vi "MXA_FSM_SweeptSA.vi"() -> ()   [LabVIEW 2021]
uses:
  MXA_TypeofMeasurment_Control.ctl
  MXA_FSM_Control.ctl
  <vilib>/Utility/error.llb/DialogType.ctl
  Control 2.ctl
  Control 3.ctl
  Control 4.ctl
  Keysight XSAn/Keysight XSAn.lvlib
panel:
  in  "ON/OFF TRIGGER":bool
  out "Power_in(mW) 2":dbl
  in  "Reset SA":bool
  out "Error SA":errorcluster
  out "Error Power Meter 2":errorcluster
  out "NewVal 2":bool
  out "Power_out(mW)":dbl
  out "Power Meter out":dbl[](graph)
  out "Power Meter Out":bool
  in  "Power Meter Out":refnum<visa-resource-name>="PM100D" caption="resource name"
  out "Power Meter in":dbl[](graph)
  in  "Power Meter In":refnum<visa-resource-name>="PM100D" caption="resource name"
  out "Power Meter In":bool
  in  "Reset Power Meter":bool
  out "Power_in(mW)":dbl
  out "NewVal":bool
  out "Error Power Meter":errorcluster
  in  "file (use dialog)":path
  in  "Base Name":string
  in  "ExternalTriggerLevel":dbl=1.0 caption="Ex_Trig_Level"
  out "Measurement Type":T1=enum."S-Meas"
  in  "Type of Normalization":enum32{"(S-N)/(N-E)", "(S-E)/(E)"}(radio)=enum."(S-E)/(E)"
  out "XY-Graph":cluster{"Val":dbl[], "Val":dbl[]}(graph)
  in  "S measurement":bool
  in  "N measurement":bool
  in  "E measurement":bool
  in  "Averages":i32
  in  "span":dbl=1000.0 caption="span (MHz)"
  in  "center frequency":dbl=520.0 caption="center frequency (MHz)"
  in  "Spectrum analyzer":string="TCPIP0::K-N9020B-50216::inst0::INSTR" caption="resource name"
  in  "stop":bool
  # "Triggering"
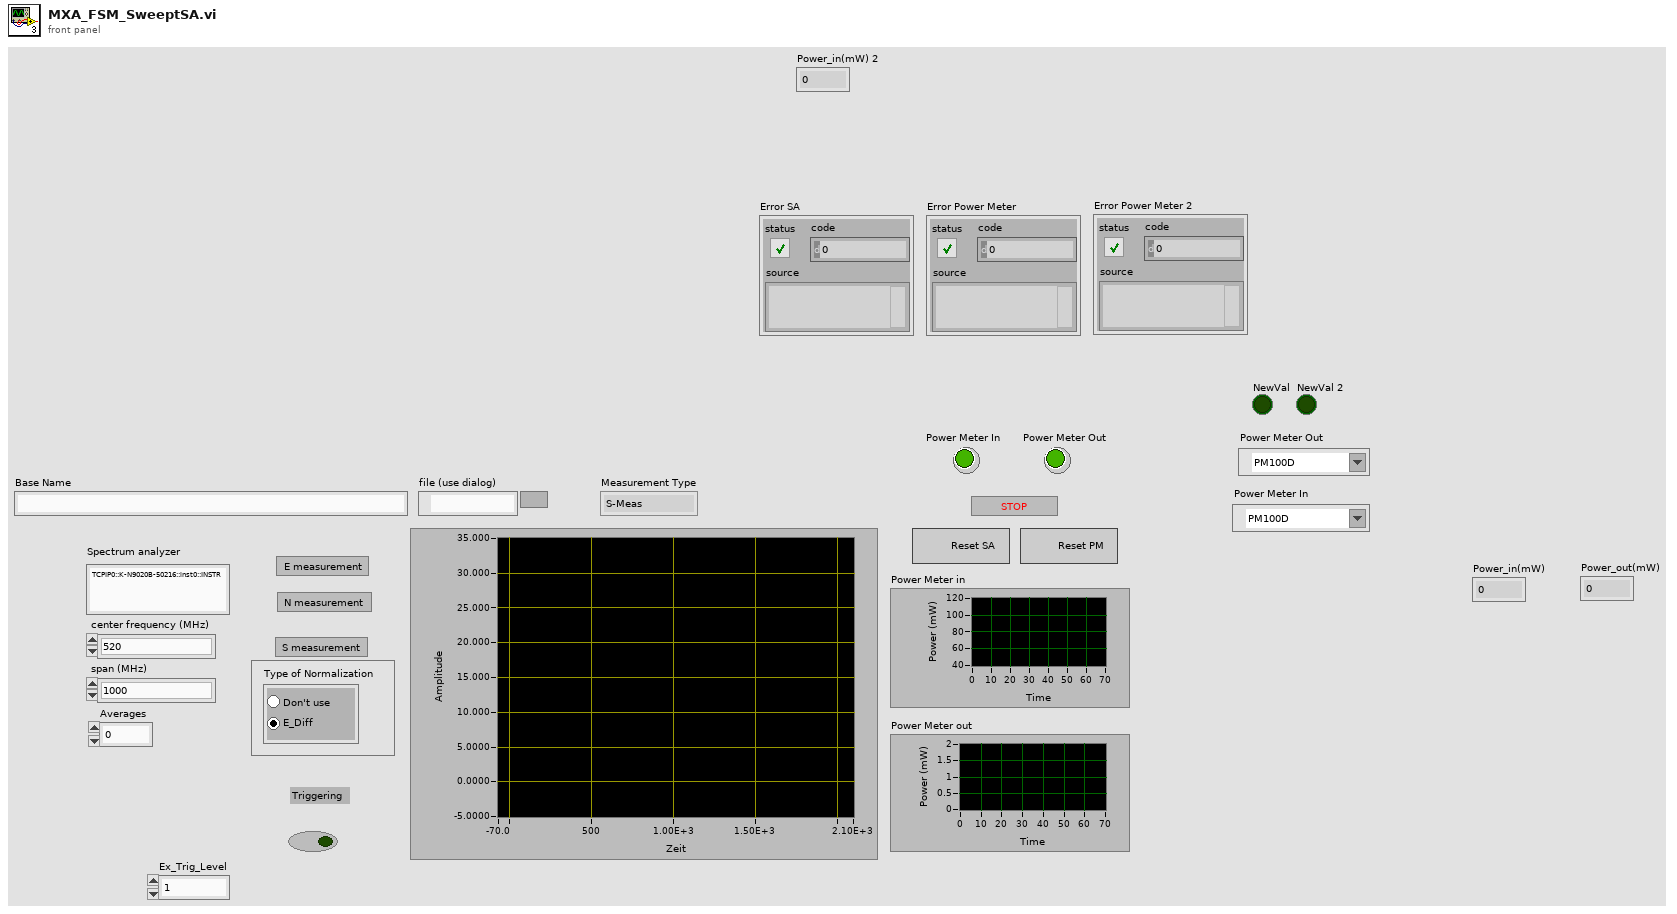
[diagram p1: front panel]
types:
  T1 = typedef "MXA_TypeofMeasurment_Control.ctl" = enum16{"N-Meas", "S-Meas", "E-Meas", "Av_S vs Power"}
  T2 = typedef "MXA_FSM_Control.ctl" = enum16{"Init", "Meas", "Run", "Exit"}
  T3 = typedef "Control 3.ctl" = path
  T4 = typedef "Control 2.ctl" = path
  T5 = typedef "Control 4.ctl" = path
  T6 = typedef "DialogType.ctl" = u16
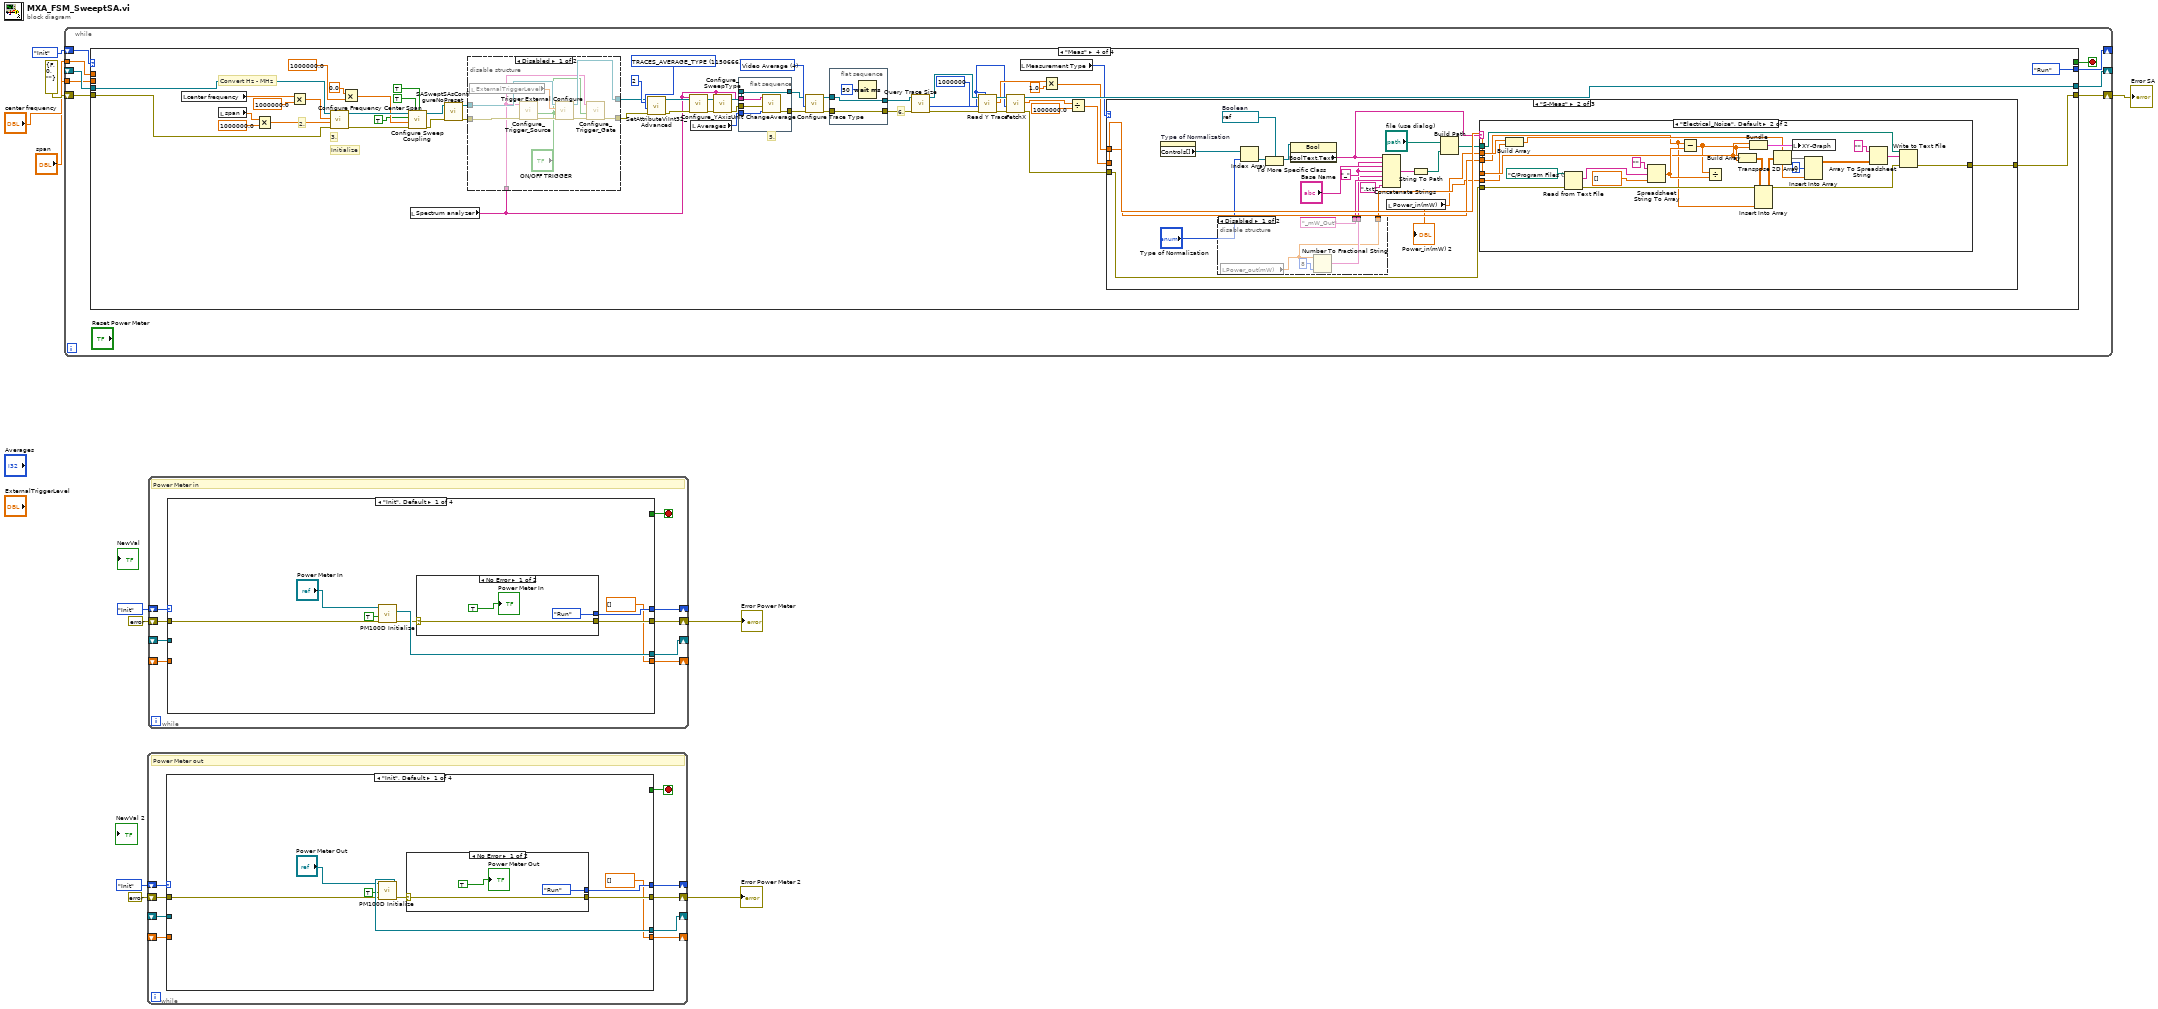
[diagram p0: block diagram]
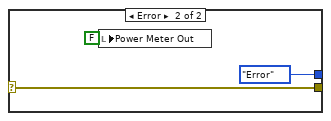
[diagram p2: hidden frame]
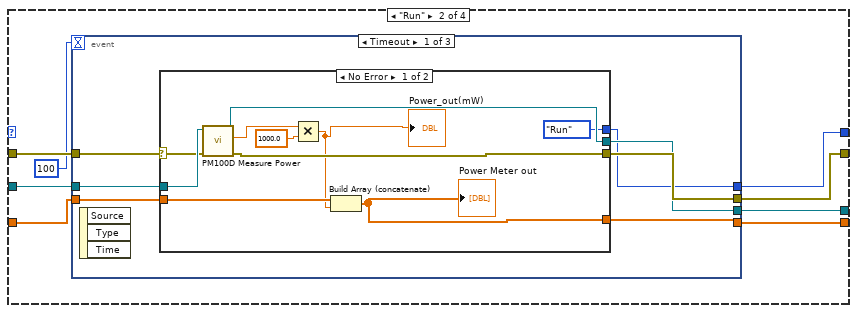
[diagram p3: hidden frame]
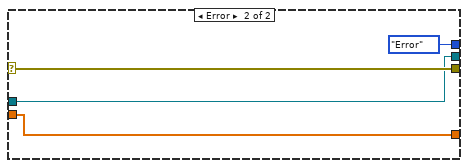
[diagram p4: hidden frame]
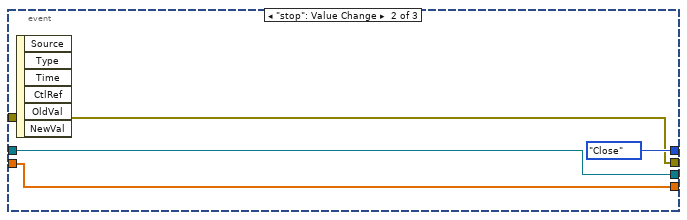
[diagram p5: hidden frame]
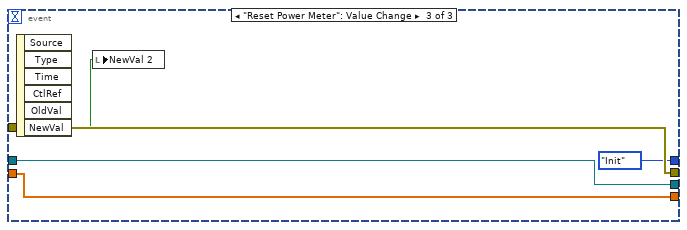
[diagram p6: hidden frame]
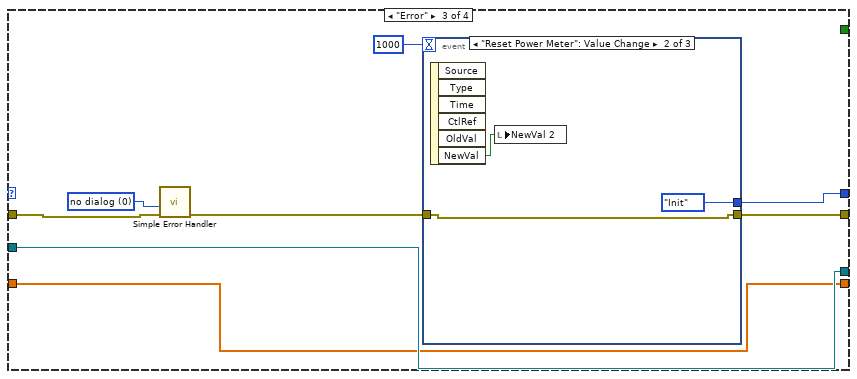
[diagram p7: hidden frame]
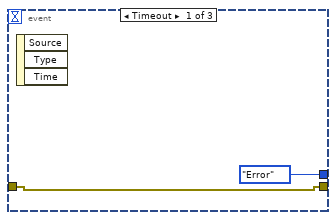
[diagram p8: hidden frame]
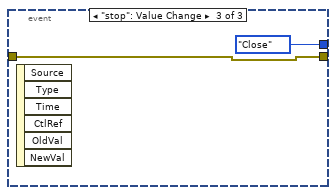
[diagram p9: hidden frame]
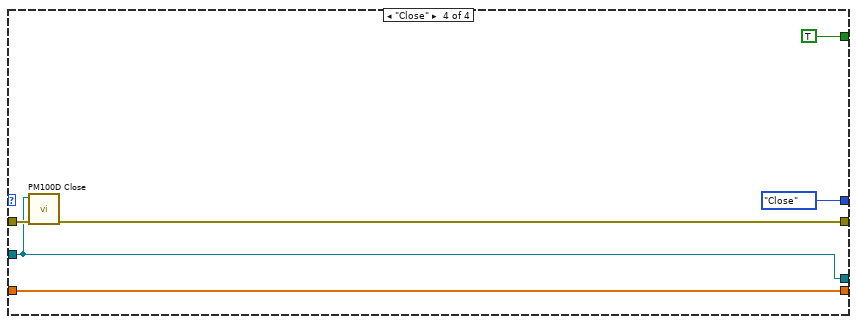
[diagram p10: hidden frame]
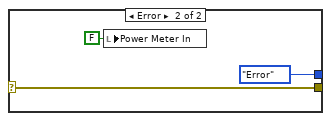
[diagram p11: hidden frame]
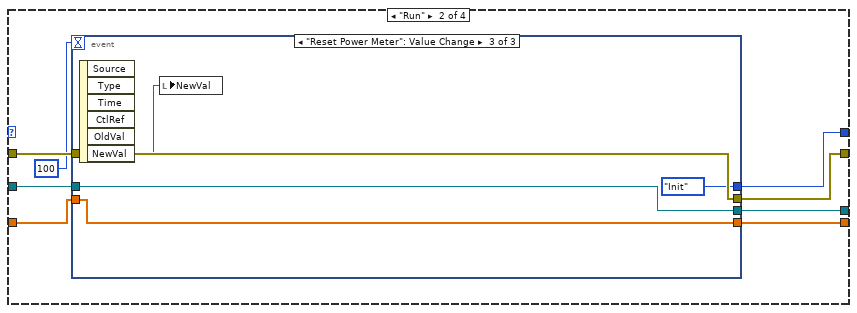
[diagram p12: hidden frame]
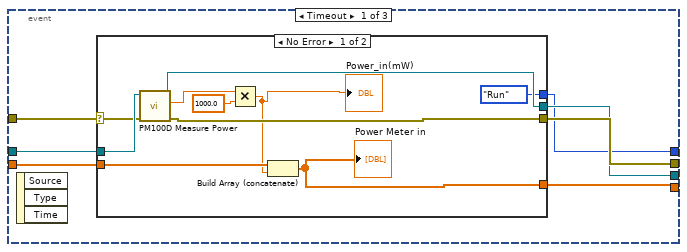
[diagram p13: hidden frame]
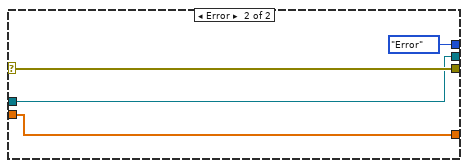
[diagram p14: hidden frame]
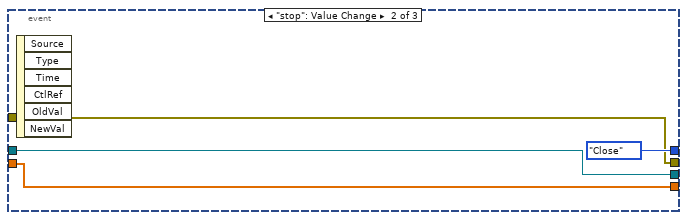
[diagram p15: hidden frame]
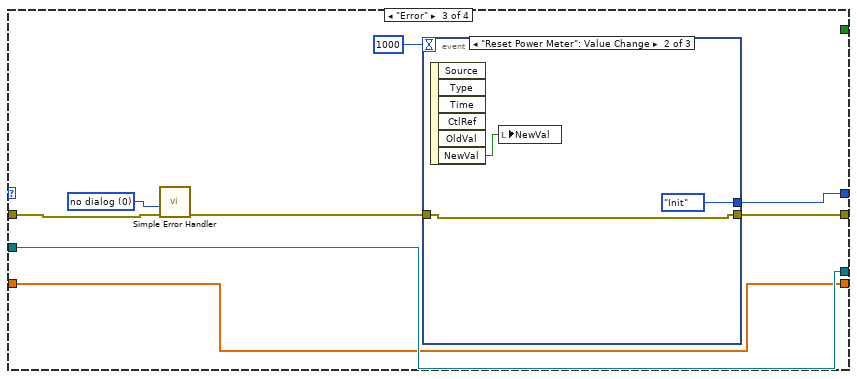
[diagram p16: hidden frame]
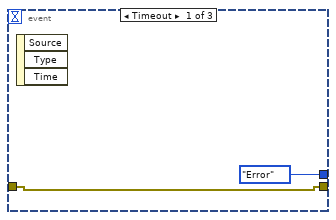
[diagram p17: hidden frame]
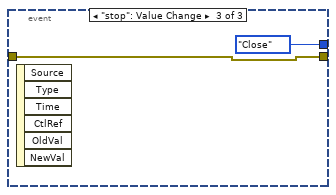
[diagram p18: hidden frame]
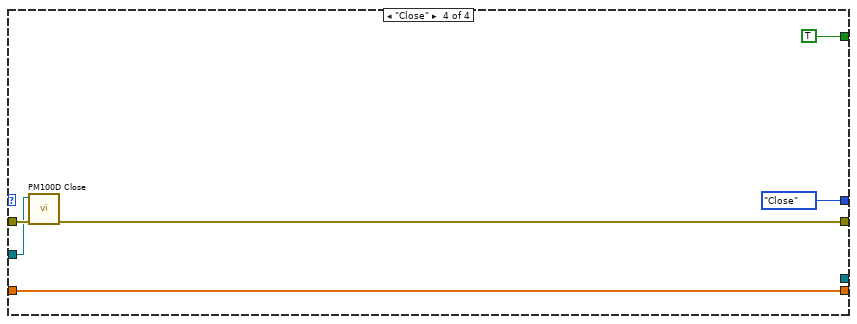
[diagram p19: hidden frame]
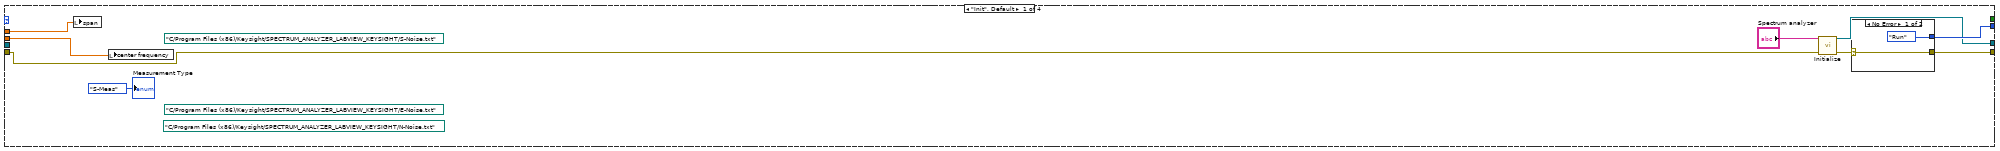
[diagram p20: hidden frame]
diagram:
  n1 = while {
    shift-right: [w19] -> _
    shift-left: MXA_FSM_Control."Init" -> [w20]
    shift-right: [w17] -> _
    shift-left: _ -> [w16]
    shift-right: [w14] -> w4
    shift-left: errorcluster {"status"=FALSE, "code"=0, "source"=""} ("error in (no error)") -> [w15]
    tunnel: "center frequency" -> [w13]
    tunnel: "span" -> [w12]
    stop <- w18 stop-if-true
    n2 = case shown="\"Meas\"" w20 {
      tunnel: [w29 w39 MXA_FSM_Control."Init" MXA_FSM_Control."Run"] -> w19
      tunnel: [_ _ TRUE _] -> w18
      tunnel: [w27 w36 w64 w88] -> w17
      tunnel: w16 -> [_ w37 w64 w90]
      tunnel: w15 -> [w26 w35 w62 w89]
      tunnel: [w24 w34 w63 w118] -> w14
      tunnel: w13 -> [w23 _ _ _]
      tunnel: w12 -> [w22 _ _ _]
      frame "Init", Default {
        (unwired) T5 path "C:/Program Files (x86)/Keysight/SPECTRUM_ANALYZER_LABVIEW_KEYSIGHT/S-Noise.txt" ("file (use dialog)")
        (unwired) T3 path "C:/Program Files (x86)/Keysight/SPECTRUM_ANALYZER_LABVIEW_KEYSIGHT/N-Noise.txt" ("file (use dialog)")
        (unwired) T4 path "C:/Program Files (x86)/Keysight/SPECTRUM_ANALYZER_LABVIEW_KEYSIGHT/E-Noise.txt" ("file (use dialog)")
        n3 = local write "span"(w22) -> ()
        n4 = local write "center frequency"(w23) -> ()
        n5 = call "Initialize.vi"("error in (no error)"=w26, "resource string"="Spectrum analyzer") -> ("error out"=w25:errorcluster, "instrument handle out"=w27:refnum<k15>)  [unwired: 8 in]
        n6 = case shown="No Error" w25 {
          selector: w25 -> [w31 w33]
          tunnel: [MXA_FSM_Control."Run" MXA_FSM_Control."Exit"] -> w29
          tunnel: [w31 w33] -> w24
          frame No Error {
          }
          frame Error {
          }
        }
        "Measurement Type" <- MXA_TypeofMeasurment_Control."S-Meas" ("Measurement Type")
      }
      frame "Run" {
        n7 = event shown="[2] \"Reset SA\": Value Change" {
          selector: _ -> [_ _ _ _ _ _]
          dyn-events: _ -> [_ _ _ _ _ _]
          timeout: 100 -> [_ _ _ _ _ _]
          tunnel: [MXA_FSM_Control."Run" MXA_FSM_Control."Exit" MXA_FSM_Control."Init" MXA_FSM_Control."Meas" MXA_FSM_Control."Meas" MXA_FSM_Control."Meas"] -> w39
          tunnel: w37 -> [w42 w45 w48 w52 w56 w60]
          tunnel: [w42 w45 w48 w52 w56 w60] -> w36
          tunnel: w35 -> [w41 w44 w47 w51 w55 w59]
          tunnel: [w41 w44 w47 w51 w55 w59] -> w34
          event Timeout {
            n8 = event-data() -> ()  [unwired: 1 in, 3 out]
          }
          event "stop": Value Change {
            n9 = event-data() -> ()  [unwired: 1 in, 5 out]
          }
          event "Reset SA": Value Change {
            n10 = event-data() -> ()  [unwired: 1 in, 5 out]
          }
          event "E measurement": Value Change {
            n11 = event-data() -> ()  [unwired: 1 in, 5 out]
            n12 = local write "Measurement Type"(MXA_TypeofMeasurment_Control."E-Meas" ("Measurement Type")) -> ()
          }
          event "N measurement": Value Change {
            n13 = event-data() -> ()  [unwired: 1 in, 5 out]
            n14 = local write "Measurement Type"(MXA_TypeofMeasurment_Control."N-Meas" ("Measurement Type")) -> ()
          }
          event "S measurement": Value Change {
            n15 = event-data() -> ()  [unwired: 1 in, 5 out]
            n16 = local write "Measurement Type"(MXA_TypeofMeasurment_Control."S-Meas" ("Measurement Type")) -> ()
          }
        }
      }
      frame "Exit" {
        n17 = call "Close.vi"("error in (no error)"=w62, "instrument handle"=w64) -> ("error out"=w63:errorcluster)  [unwired: 9 in]
      }
      frame "Meas" {
        w103 = u32 1150666 items=["IVILXISYNC_ARM_ALARM_REPEAT_COUNT"=1950004, "IVILXISYNC_ARM_COUNT"=1950007, "IVILXISYNC_ARM_SOURCE_DETECTION"=1950010, "IVILXISYNC_EVENT_DRIVE_MODE"=1950030, "IVILXISYNC_EVENT_SLOPE"=1950031, "IVILXISYNC_EVENT_WIRED_OR_BIAS_MODE"=1950033, "IVILXISYNC_TRIGGER_ALARM_REPEAT_COUNT"=1950018, "IVILXISYNC_TRIGGER_COUNT"=1950021, "IVILXISYNC_TRIGGER_SOURCE_DETECTION"=1950025, "LEVEL_ATTENUATION_OPTIMIZE"=1150012, "LEVEL_ATTENUATION_STEP_INCREMENT"=1150013, "LEVEL_ELECTRONIC_ATTENUATION"=1150578, "MEMORYOPERATION_SCREEN_IMAGE_THEME"=1150678, "NUMBER_OF_SWEEPS"=1250010, "OUTPUT_ANALOG_TYPE"=1150679, "OUTPUT_AUXILIARY_IF_TYPE"=1150681, "PRESELECTOR_MW_PATH"=1150585, "RADIO_BAND_CLASS"=1150550, "RADIO_DEVICE"=1150547, "RADIO_NON_STANDARD_MEASUREMENT_ENABLED"=1150549, "RADIO_PACKET_TYPE"=1150551, "RADIO_STANDARD"=1150548, "REFOSCILLATOR_EXTERNAL_BANDWIDTH"=1150539, "REFOSCILLATOR_EXTERNAL_COUPLING"=1150538, "REFOSCILLATOR_SOURCE "=1150877, "STATETRIGGER_DETECTION"=1150159, "SYSTEM_IO_TIMEOUT"=1150783, "SYSTEM_TIMEOUT_MILLISECONDS"=1150175, "TRACE_DETECTOR_TYPE"=1150782, "TRACE_TYPE"=1250020, "TRACES_AVERAGE_TYPE"=1150666, "TRIGGER_EXTERNAL2_SLOPE"=1150671, "TRIGGER_EXTERNAL_SLOPE"=1150803, "TRIGGER_FRAME_SYNC_SOURCE"=1150841, "TRIGGER_LINE_DELAY_SLOPE"=1150836, "TRIGGER_RFBURST_SLOPE "=1150830, "TRIGGER_SOURCE"=1250301, "TRIGGER_VIDEO_SLOPE"=1150806, "VERTICAL_SCALE"=1250021, "VIDEO_TRIGGER_SLOPE"=1250502] ("AttributeID")
        w104 = 4 items=["Clear Write"=1, "Maximum Hold"=2, "Minimum Hold"=3, "Video Average"=4, "View"=5, "Store"=6] ("trace type (Clear Write)")
        # "Convert Hz - MHz"
        # "3."
        # "2."
        # "6."
        # "5."
        # "Initialize"
        n18 = local read "center frequency"() -> (w93:dbl)
        n19 = local read "span"() -> (w92:dbl)
        n20 = Multiply(x=w92, y=1000000.0) -> (x*y=w112:dbl)
        n21 = Multiply(x=w93, y=1000000.0) -> (x*y=w114:dbl)
        n22 = call "Configure Frequency Center Span.vi"("error in (no error)"=w89, "span"=w112, "center frequency"=w114, "instrument handle"=w90) -> ("error out"=w116:errorcluster, "instrument handle out"=w117:refnum<k15>)  [unwired: 6 in]
        n23 = Multiply(x=0.0, y=1000000.0) -> (x*y=w110:dbl)
        n24 = call "Configure Sweep Coupling.vi"("sweep time auto (Off)"=TRUE, "video bandwidth auto (Off)"=TRUE, "error in (no error)"=w116, "resolution bandwidth"=w110, "resolution bandwidth auto (Off)"=TRUE, "instrument handle"=w117) -> ("error out"=w107:errorcluster, "instrument handle out"=w108:refnum<k15>)  [unwired: 4 in]
        n25 = local read "Spectrum analyzer"() -> (w66:string)
        n26 = call "SASweptSAsConfigureNoPreset.vi"("error in (no error)"=w107, "instrument handle"=w108) -> ("error out"=w68:errorcluster, "instrument handle out"=w70:refnum<k15>)  [unwired: 8 in]
        n27 = disable-structure shown="Disabled" {
          disable-tunnel: w70 -> [w128 w130]
          disable-tunnel: [w127 w130] -> w69
          disable-tunnel: w68 -> [w125 w129]
          disable-tunnel: [w122 w129] -> w67
          disable-tunnel: w66 -> [w121 _]
          frame Disabled {
            n28 = local read "ExternalTriggerLevel"() -> (w126:dbl)
            n29 = call "Configure_Trigger_Source.vi"("error in (no error)"=w125, "ON/OFF TRIGGER"="ON/OFF TRIGGER", "VISA resource name"=w121) -> ("error out"=w124:errorcluster)  [unwired: 7 in, 1 out]
            n30 = call "Trigger External Configure.vi"("error in (no error)"=w124, "ExternalTriggerLevel"=w126, "instrument handle"=w128) -> ("error out"=w123:errorcluster, "instrument handle out"=w127:refnum<k15>)  [unwired: 7 in]
            n31 = call "Configure_Trigger_Gate.vi"("error in (no error)"=w123, "ON/OFF TRIGGER"="ON/OFF TRIGGER", "VISA resource name"=w121) -> ("error out"=w122:errorcluster)  [unwired: 8 in]
          }
          frame Enabled {
          }
        }
        n32 = call "SetAttributeViInt32_Advanced.vi"("AttributeValue"=2, "error in (no error)"=w67, "AttributeID"=w103, "instrument handle"=w69) -> ("error out"=w78:errorcluster, "instrument handle out"=w100:refnum<k15>)  [unwired: 6 in]
        n33 = call "Configure_YAxisUnit.vi"("error in (no error)"=w78, "VISA resource name"=w66) -> ("error out"=w77:errorcluster)  [unwired: 9 in]
        n34 = local read "Averages"() -> (w91:i32)
        n35 = call "Configure_SweepType.vi"("error in (no error)"=w77, "VISA resource name"=w66) -> ("error out"=w87:errorcluster)  [unwired: 9 in]
        n36 = flat-sequence {
          tunnel: w87 -> [w135]
          tunnel: [w134] -> w101
          tunnel: w66 -> [w133]
          tunnel: w91 -> [w132]
          tunnel: w100 -> [w131]
          tunnel: [w131] -> w99
          frame #0 {
            n37 = call "ChangeAverage.vi"("Averages"=w132, "error in (no error)"=w135, "VISA resource name"=w133) -> ("error out"=w134:errorcluster)  [unwired: 8 in]
          }
        }
        n38 = call "Configure Trace Type.vi"("error in (no error)"=w101, "trace type (Clear Write)"=w104, "instrument handle"=w99) -> ("error out"=w105:errorcluster, "instrument handle out"=w106:refnum<k15>)  [unwired: 7 in]
        n39 = flat-sequence {
          tunnel: w106 -> [w137]
          tunnel: [w137] -> w76
          tunnel: w105 -> [w136]
          tunnel: [w136] -> w75
          frame #0 {
            n40 = Wait (ms)(milliseconds to wait=u32 50) -> ()  [unwired: 1 out]
          }
        }
        n41 = call "Query Trace Size.vi"("error in (no error)"=w75, "instrument handle"=w76) -> ("error out"=w74:errorcluster, "trace size"=w72:i32, "instrument handle out"=w73:refnum<k15>)  [unwired: 7 in]
        n42 = call "Read Y Trace.vi"("array length"=w72, "error in (no error)"=w74, "maximum time"=1000000, "instrument handle"=w73) -> ("error out"=w96:errorcluster, "amplitude"=w80:dbl[], "instrument handle out"=w97:refnum<k15>)  [unwired: 4 in, 1 out]
        n43 = call "FetchX.vi"("error in (no error)"=w96, "ValBufferSize"=w72, "instrument handle"=w97) -> ("error out"=w83:errorcluster, "Val"=w95:dbl[], "instrument handle out"=w88:refnum<k15>)  [unwired: 5 in, 1 out]
        n44 = local read "Measurement Type"() -> (w71:T1)
        n45 = Multiply(x=w80, y=1.0) -> (x*y=w79:dbl[])
        n46 = Divide(x=w95, y=1000000.0) -> (x/y=w82:dbl[])
        n47 = case shown="\"S-Meas\"" w71 {
          tunnel: [w145 w166 w230] -> w118
          tunnel: w83 -> [w146 w167 w231]
          tunnel: w82 -> [w144 w165 w228]
          tunnel: w79 -> [w141 w164 w226]
          frame "N-Meas", Default {
            n48 = Bundle(w144, w141) -> (w143:cluster{dbl[], dbl[]})  [unwired: 1 in]
            n49 = Array To Spreadsheet String(array=w141, 3:"") -> (spreadsheet string=w140:string)  [unwired: 1 in]
            n50 = local write "XY-Graph"(w143) -> ()
            n51 = Write to Text File(file (use dialog)=T3 path "C:/Program Files (x86)/Keysight/SPECTRUM_ANALYZER_LABVIEW_KEYSIGHT/N-Noise.txt", text=w140, error in=w146) -> (error out=w145:errorcluster)  [unwired: 1 in, 2 out]
          }
          frame "S-Meas" {
            w151 = "_" ("string")
            w154 = refnum<vi> refnum  # Boolean
            n52 = property on="Type of Normalization" class="RadioBtnsControl (strict)"() -> ("Controls[]"=w156:refnum<vi>[])  [unwired: 2 in, 2 out]
            n53 = disable-structure shown="Disabled" {
              disable-tunnel: ["_mW_Out" ("string") _] -> w157
              disable-tunnel: [w170 _] -> w149
              disable-tunnel: [w168 _] -> w148
              frame Disabled {
                n54 = local read "Power_out(mW)"() -> (w168:dbl)
                n55 = Number To Fractional String(number=w168, precision (6)=i16 8) -> (F-format string=w170:string)  [unwired: 2 in]
              }
              frame Enabled {
              }
            }
            n56 = Index Array(array=w156, index="Type of Normalization") -> (element=w155:refnum<vi>)
            n57 = To More Specific Class(target class=w154, reference=w155) -> (specific class reference=w153:refnum<vi>)  [unwired: 1 in, 1 out]
            n58 = property class="Bool"(reference=w153) -> ("BoolText.Text"=w150:string)  [unwired: 1 in, 2 out]
            n59 = Concatenate Strings(w150, w151, "Base Name", w151, w149, w157, ".txt" ("string")) -> (w161:string)
            n60 = local read "Power_in(mW)"() -> (w147:dbl)
            "Power_in(mW) 2" <- w147
            n61 = String To Path(string=w161) -> (path=w159:path)
            n62 = Build Path(base path="file (use dialog)", name or relative path=w159) -> (appended path=w158:path)
            n63 = case shown="\"Electrical_Noise\", Default" w150 {
              tunnel: w167 -> [w200 w223]
              tunnel: [w181 w213] -> w166
              tunnel: w165 -> [w184 w215]
              tunnel: w164 -> [w194 w203]
              tunnel: w158 -> [w178 w211]
              tunnel: w147 -> [w175 w210]
              tunnel: w148 -> [w174 w209]
              frame "Shot_Noise" {
                n64 = Read from Text File(file (use dialog)=T4 path "C:/Program Files (x86)/Keysight/SPECTRUM_ANALYZER_LABVIEW_KEYSIGHT/E-Noise.txt", error in=w200) -> (text=w197:string, error out=w199:errorcluster)  [unwired: 2 in, 2 out]
                n65 = Read from Text File(file (use dialog)=T3 path "C:/Program Files (x86)/Keysight/SPECTRUM_ANALYZER_LABVIEW_KEYSIGHT/N-Noise.txt", error in=w199) -> (text=w195:string, error out=w182:errorcluster)  [unwired: 2 in, 2 out]
                n66 = Spreadsheet String To Array(format string="", spreadsheet string=w197, array type (2D Dbl)=dbl[] [] ("amplitude")) -> (array=w192:dbl[])  [unwired: 1 in]
                n67 = Spreadsheet String To Array(format string="", spreadsheet string=w195, array type (2D Dbl)=dbl[] [] ("amplitude")) -> (array=w193:dbl[])  [unwired: 1 in]
                n68 = Subtract(x=w194, y=w193) -> (x-y=w191:dbl[])
                n69 = Subtract(x=w193, y=w192) -> (x-y=w190:dbl[])
                n70 = Build Array(w175, w174) -> (w177:dbl[])
                n71 = Divide(x=w191, y=w190) -> (x/y=w183:dbl[])
                n72 = Bundle(w184, w183) -> (w189:cluster{dbl[], dbl[]})  [unwired: 1 in]
                n73 = Build Array(w184, w183) -> (w173:dbl[][])
                n74 = local write "XY-Graph"(w189) -> ()
                n75 = Insert Into Array(array=w173, new element=w177) -> (w176:dbl[][])  [unwired: 2 in]
                n76 = Transpose 2D Array(2D array=w176) -> (transposed array=w172:dbl[][])
                n77 = Array To Spreadsheet String(array=w172, 3:"") -> (spreadsheet string=w185:string)  [unwired: 1 in]
                n78 = Write to Text File(file (use dialog)=w178, text=w185, error in=w182) -> (error out=w181:errorcluster)  [unwired: 1 in, 2 out]
              }
              frame "Electrical_Noise", Default {
                n79 = Build Array(w210, w209) -> (w208:dbl[])
                n80 = Read from Text File(file (use dialog)=T4 path "C:/Program Files (x86)/Keysight/SPECTRUM_ANALYZER_LABVIEW_KEYSIGHT/E-Noise.txt", error in=w223) -> (text=w222:string, error out=w214:errorcluster)  [unwired: 2 in, 2 out]
                n81 = Spreadsheet String To Array(format string="", spreadsheet string=w222, array type (2D Dbl)=dbl[] [] ("amplitude")) -> (array=w220:dbl[])  [unwired: 1 in]
                n82 = Subtract(x=w203, y=w220) -> (x-y=w201:dbl[])
                n83 = Divide(x=w201, y=w220) -> ()  [unwired: 1 out]
                n84 = Build Array(w215, w201) -> (w204:dbl[][])
                n85 = Bundle(w215, w201) -> (w219:cluster{dbl[], dbl[]})  [unwired: 1 in]
                n86 = Insert Into Array(array=w204, new element=w203) -> (w202:dbl[][])  [unwired: 2 in]
                n87 = Transpose 2D Array(2D array=w202) -> (transposed array=w207:dbl[][])
                n88 = local write "XY-Graph"(w219) -> ()
                n89 = Insert Into Array(array=w207, index (row)=0, new element=w208) -> (w205:dbl[][])  [unwired: 1 in]
                n90 = Array To Spreadsheet String(array=w205, 3:"") -> (spreadsheet string=w216:string)  [unwired: 1 in]
                n91 = Write to Text File(file (use dialog)=w211, text=w216, error in=w214) -> (error out=w213:errorcluster)  [unwired: 1 in, 2 out]
              }
            }
          }
          frame "E-Meas" {
            n92 = Bundle(w228, w226) -> (→"XY-Graph":cluster{dbl[], dbl[]})  [unwired: 1 in]
            n93 = Array To Spreadsheet String(array=w226, 3:"") -> (spreadsheet string=w225:string)  [unwired: 1 in]
            n94 = Write to Text File(file (use dialog)=T4 path "C:/Program Files (x86)/Keysight/SPECTRUM_ANALYZER_LABVIEW_KEYSIGHT/E-Noise.txt", text=w225, error in=w231) -> (error out=w230:errorcluster)  [unwired: 1 in, 2 out]
          }
        }
      }
    }
  }
  "Error SA" <- w4
  n95 = while {
    shift-right: [w239] -> _
    shift-left: _ -> [w236]
    shift-right: [w238] -> _
    shift-left: enum16{"Init", "Run", "Error", "Close"}."Init" -> [w240]
    shift-right: [w237] -> w3
    shift-left: errorcluster {"status"=FALSE, "code"=0, "source"=""} ("error out") -> [w235]
    shift-right: [w232] -> _
    shift-left: _ -> [w233]
    stop <- w234 stop-if-true
    # "Power Meter out"
    n96 = case shown="\"Init\", Default" w240 {
      tunnel: [w248 w261 w298 w308] -> w239
      tunnel: [w246 w262 w296 enum16{"Init", "Run", "Error", "Close"}."Close"] -> w238
      tunnel: [w247 w260 w295 w311] -> w237
      tunnel: w236 -> [_ w258 w298 w308]
      tunnel: w235 -> [w245 w259 w300 w312]
      tunnel: [_ _ _ TRUE] -> w234
      tunnel: w233 -> [_ w256 w297 w309]
      tunnel: [dbl[] [] w255 w297 w309] -> w232
      frame "Init", Default {
        n97 = call "PM100D Initialize.vi"("error in (no error)"=w245, "Reset Device (Reset Device)"=TRUE, "resource name"="Power Meter Out") -> ("error out"=w243:errorcluster, "instrument handle out"=w248:refnum<visa-resource-name>)  [unwired: 7 in]
        n98 = case shown="No Error" w243 {
          selector: w243 -> [w251 w253]
          tunnel: [w251 w253] -> w247
          tunnel: [enum16{"Init", "Run", "Error", "Close"}."Run" enum16{"Init", "Run", "Error", "Close"}."Error"] -> w246
          frame No Error {
            "Power Meter Out" <- TRUE ("Power Meter")
          }
          frame Error {
            n99 = local write "Power Meter Out"(FALSE ("Power Meter")) -> ()
          }
        }
      }
      frame "Run" {
        n100 = event shown="[0] Timeout" {
          selector: _ -> [_ _ _]
          dyn-events: _ -> [_ _ _]
          timeout: 100 -> [_ _ _]
          tunnel: [w263 enum16{"Init", "Run", "Error", "Close"}."Close" enum16{"Init", "Run", "Error", "Close"}."Init"] -> w262
          tunnel: [w267 w286 w291] -> w261
          tunnel: [w268 w285 w292] -> w260
          tunnel: w259 -> [w264 w285 w292]
          tunnel: w258 -> [w269 w286 w291]
          tunnel: w256 -> [w266 w284 w290]
          tunnel: [w265 w284 w290] -> w255
          event Timeout {
            n101 = event-data() -> ()  [unwired: 1 in, 3 out]
            n102 = case shown="No Error" w264 {
              selector: w264 -> [w272 w282]
              tunnel: w269 -> [w279 w281]
              tunnel: [w278 w282] -> w268
              tunnel: [w277 w281] -> w267
              tunnel: w266 -> [w276 w283]
              tunnel: [w275 w283] -> w265
              tunnel: [enum16{"Init", "Run", "Error", "Close"}."Run" enum16{"Init", "Run", "Error", "Close"}."Error"] -> w263
              frame No Error {
                n103 = call <instrlib>:"PM100D Measure Power.vi"("error in (no error)"=w272, "instrument handle"=w279) -> ("error out"=w278:errorcluster, "Power"=w274:dbl, "instrument handle out"=w277:refnum<visa-resource-name>)  [unwired: 7 in]
                n104 = Multiply(x=w274, y=1000.0) -> (x*y=w270:dbl)
                "Power_out(mW)" <- w270
                n105 = Build Array (concatenate)(w276, w270) -> (w275:dbl[])
                "Power Meter out" <- w275
              }
              frame Error {
              }
            }
          }
          event "stop": Value Change {
            n106 = event-data() -> ()  [unwired: 1 in, 6 out]
          }
          event "Reset Power Meter": Value Change {
            n107 = event-data() -> ("NewVal"=w288:bool)  [unwired: 1 in, 5 out]
            n108 = local write "NewVal 2"(w288) -> ()
          }
        }
      }
      frame "Error" {
        w299 = T6 0 items=["no dialog", "OK message", "continue or stop message", "OK message + warnings", "continue/stop + warnings"] ("type of dialog (OK msg:1)")
        n109 = call <vilib>:"Simple Error Handler.vi"("type of dialog (OK msg:1)"=w299, "error in (no error)"=w300) -> ("error out"=w294:errorcluster)  [unwired: 3 in, 4 out]
        n110 = event shown="[1] \"Reset Power Meter\": Value Change" {
          selector: _ -> [_ _ _]
          dyn-events: _ -> [_ _ _]
          timeout: 1000 -> [_ _ _]
          tunnel: [enum16{"Init", "Run", "Error", "Close"}."Error" enum16{"Init", "Run", "Error", "Close"}."Init" enum16{"Init", "Run", "Error", "Close"}."Close"] -> w296
          tunnel: [w301 w304 w306] -> w295
          tunnel: w294 -> [w301 w304 w306]
          event Timeout {
            n111 = event-data() -> ()  [unwired: 1 in, 3 out]
          }
          event "Reset Power Meter": Value Change {
            n112 = event-data() -> ("NewVal"=w303:bool)  [unwired: 1 in, 5 out]
            n113 = local write "NewVal 2"(w303) -> ()
          }
          event "stop": Value Change {
            n114 = event-data() -> ()  [unwired: 1 in, 6 out]
          }
        }
      }
      frame "Close" {
        n115 = call "PM100D Close.vi"("error in (no error)"=w312, "instrument handle"=w308) -> ("error out"=w311:errorcluster)  [unwired: 9 in]
      }
    }
  }
  "Error Power Meter 2" <- w3
  n116 = while {
    shift-right: [w321] -> _
    shift-left: _ -> [w318]
    shift-right: [w320] -> _
    shift-left: enum16{"Init", "Run", "Error", "Close"}."Init" -> [w322]
    shift-right: [w319] -> w7
    shift-left: errorcluster {"status"=FALSE, "code"=0, "source"=""} ("error out") -> [w317]
    shift-right: [w314] -> _
    shift-left: _ -> [w315]
    stop <- w316 stop-if-true
    # "Power Meter in"
    n117 = case shown="\"Init\", Default" w322 {
      tunnel: [w330 w343 w380 _] -> w321
      tunnel: [w328 w344 w378 enum16{"Init", "Run", "Error", "Close"}."Close"] -> w320
      tunnel: [w329 w342 w377 w393] -> w319
      tunnel: w318 -> [_ w340 w380 w390]
      tunnel: w317 -> [w327 w341 w382 w394]
      tunnel: [_ _ _ TRUE] -> w316
      tunnel: w315 -> [_ w338 w379 w391]
      tunnel: [dbl[] [] w337 w379 w391] -> w314
      frame "Init", Default {
        n118 = call "PM100D Initialize.vi"("error in (no error)"=w327, "Reset Device (Reset Device)"=TRUE, "resource name"="Power Meter In") -> ("error out"=w325:errorcluster, "instrument handle out"=w330:refnum<visa-resource-name>)  [unwired: 7 in]
        n119 = case shown="No Error" w325 {
          selector: w325 -> [w333 w335]
          tunnel: [w333 w335] -> w329
          tunnel: [enum16{"Init", "Run", "Error", "Close"}."Run" enum16{"Init", "Run", "Error", "Close"}."Error"] -> w328
          frame No Error {
            "Power Meter In" <- TRUE ("Power Meter")
          }
          frame Error {
            n120 = local write "Power Meter In"(FALSE ("Power Meter")) -> ()
          }
        }
      }
      frame "Run" {
        n121 = event shown="[2] \"Reset Power Meter\": Value Change" {
          selector: _ -> [_ _ _]
          dyn-events: _ -> [_ _ _]
          timeout: 100 -> [_ _ _]
          tunnel: [w345 enum16{"Init", "Run", "Error", "Close"}."Close" enum16{"Init", "Run", "Error", "Close"}."Init"] -> w344
          tunnel: [w349 w368 w373] -> w343
          tunnel: [w350 w367 w374] -> w342
          tunnel: w341 -> [w346 w367 w374]
          tunnel: w340 -> [w351 w368 w373]
          tunnel: w338 -> [w348 w366 w372]
          tunnel: [w347 w366 w372] -> w337
          event Timeout {
            n122 = event-data() -> ()  [unwired: 1 in, 3 out]
            n123 = case shown="No Error" w346 {
              selector: w346 -> [w354 w364]
              tunnel: w351 -> [w361 w363]
              tunnel: [w360 w364] -> w350
              tunnel: [w359 w363] -> w349
              tunnel: w348 -> [w358 w365]
              tunnel: [w357 w365] -> w347
              tunnel: [enum16{"Init", "Run", "Error", "Close"}."Run" enum16{"Init", "Run", "Error", "Close"}."Error"] -> w345
              frame No Error {
                n124 = call <instrlib>:"PM100D Measure Power.vi"("error in (no error)"=w354, "instrument handle"=w361) -> ("error out"=w360:errorcluster, "Power"=w356:dbl, "instrument handle out"=w359:refnum<visa-resource-name>)  [unwired: 7 in]
                n125 = Multiply(x=w356, y=1000.0) -> (x*y=w352:dbl)
                "Power_in(mW)" <- w352
                n126 = Build Array (concatenate)(w358, w352) -> (w357:dbl[])
                "Power Meter in" <- w357
              }
              frame Error {
              }
            }
          }
          event "stop": Value Change {
            n127 = event-data() -> ()  [unwired: 1 in, 6 out]
          }
          event "Reset Power Meter": Value Change {
            n128 = event-data() -> ("NewVal"=w370:bool)  [unwired: 1 in, 5 out]
            n129 = local write "NewVal"(w370) -> ()
          }
        }
      }
      frame "Error" {
        w381 = T6 0 items=["no dialog", "OK message", "continue or stop message", "OK message + warnings", "continue/stop + warnings"] ("type of dialog (OK msg:1)")
        n130 = call <vilib>:"Simple Error Handler.vi"("type of dialog (OK msg:1)"=w381, "error in (no error)"=w382) -> ("error out"=w376:errorcluster)  [unwired: 3 in, 4 out]
        n131 = event shown="[1] \"Reset Power Meter\": Value Change" {
          selector: _ -> [_ _ _]
          dyn-events: _ -> [_ _ _]
          timeout: 1000 -> [_ _ _]
          tunnel: [enum16{"Init", "Run", "Error", "Close"}."Error" enum16{"Init", "Run", "Error", "Close"}."Init" enum16{"Init", "Run", "Error", "Close"}."Close"] -> w378
          tunnel: [w383 w386 w388] -> w377
          tunnel: w376 -> [w383 w386 w388]
          event Timeout {
            n132 = event-data() -> ()  [unwired: 1 in, 3 out]
          }
          event "Reset Power Meter": Value Change {
            n133 = event-data() -> ("NewVal"=w385:bool)  [unwired: 1 in, 5 out]
            n134 = local write "NewVal"(w385) -> ()
          }
          event "stop": Value Change {
            n135 = event-data() -> ()  [unwired: 1 in, 6 out]
          }
        }
      }
      frame "Close" {
        n136 = call "PM100D Close.vi"("error in (no error)"=w394, "instrument handle"=w390) -> ("error out"=w393:errorcluster)  [unwired: 9 in]
      }
    }
  }
  "Error Power Meter" <- w7
